vi "Collate_Measurements v0.3.vi"(1 "Collate Files":bool) -> ()   [LabVIEW 2014]
uses:
  <vilib>/Utility/error.llb/DialogType.ctl
panel:
  out "appended array":dbl[][](array[numeric])
  out "FF":dbl
  out "VOC":dbl format="%#.6g"
  out "JSC":dbl
  out "PCE":dbl
  out "Array of File Paths":string[](array[string])
  out "error out":errorcluster
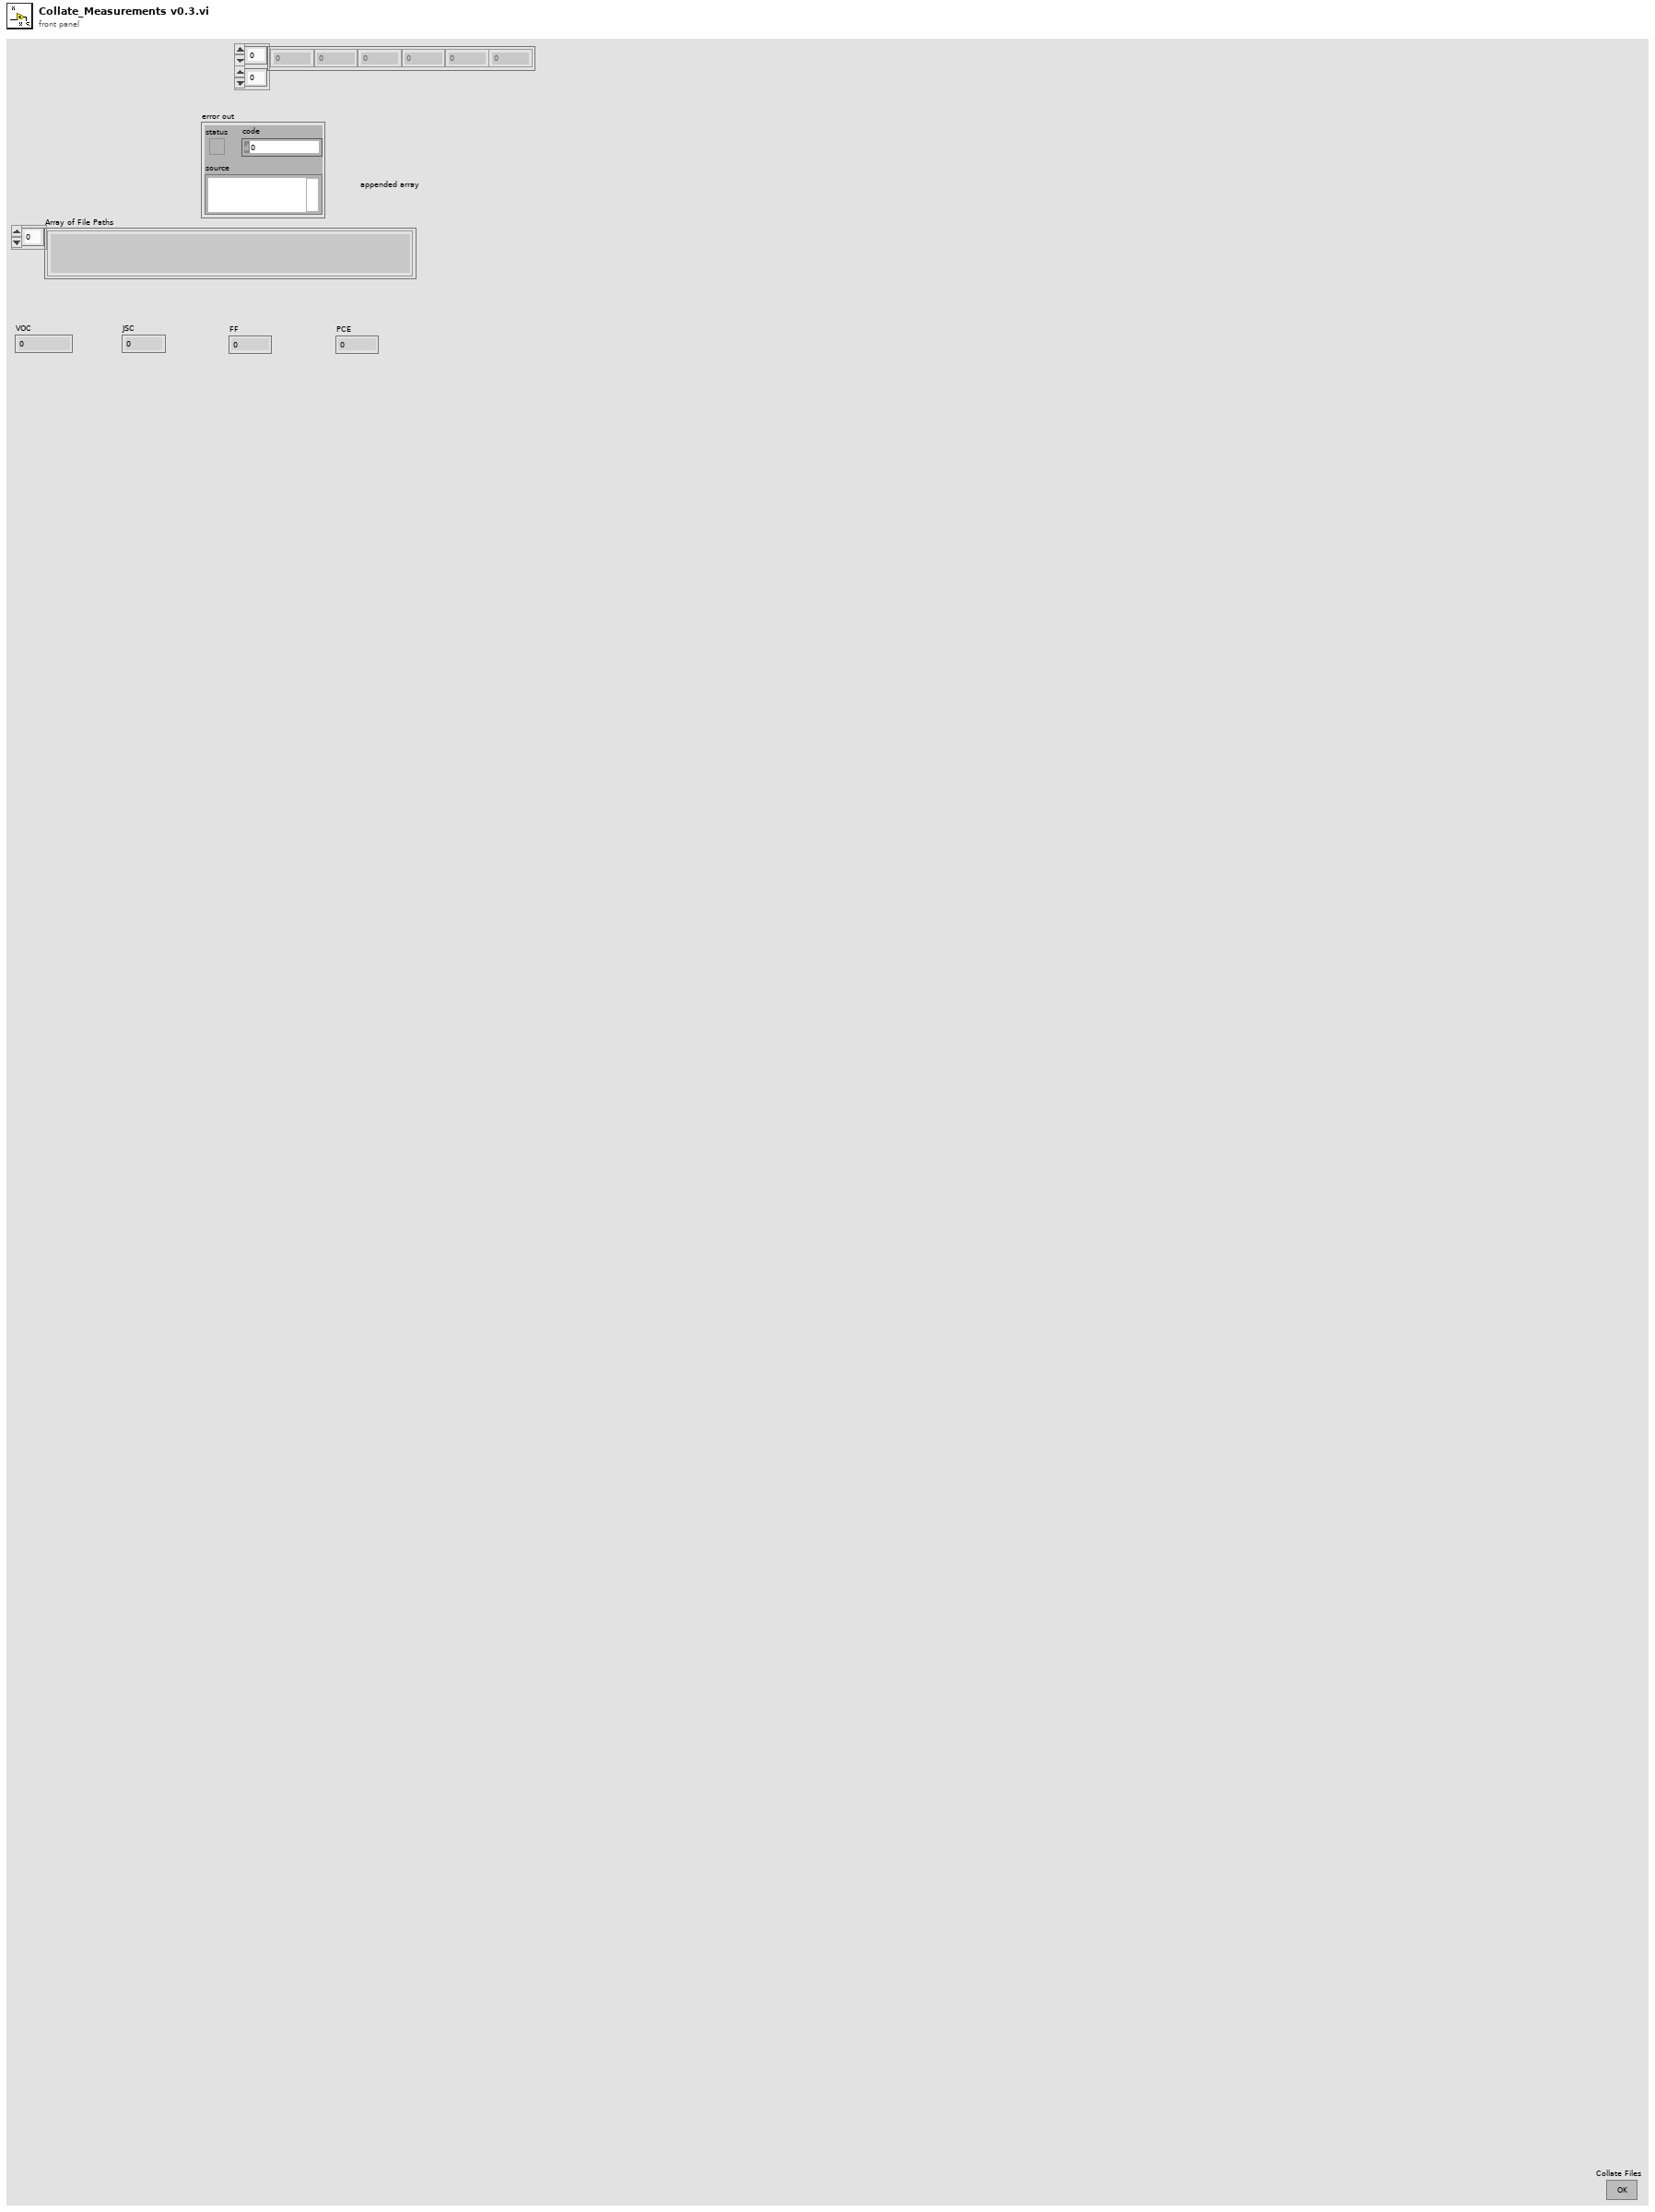
[diagram p1: front panel]
types:
  T1 = enum16{"open", "replace", "create", "open or create", "replace or create", "replace or create with confirmation"}
  T2 = typedef "DialogType.ctl" = u16
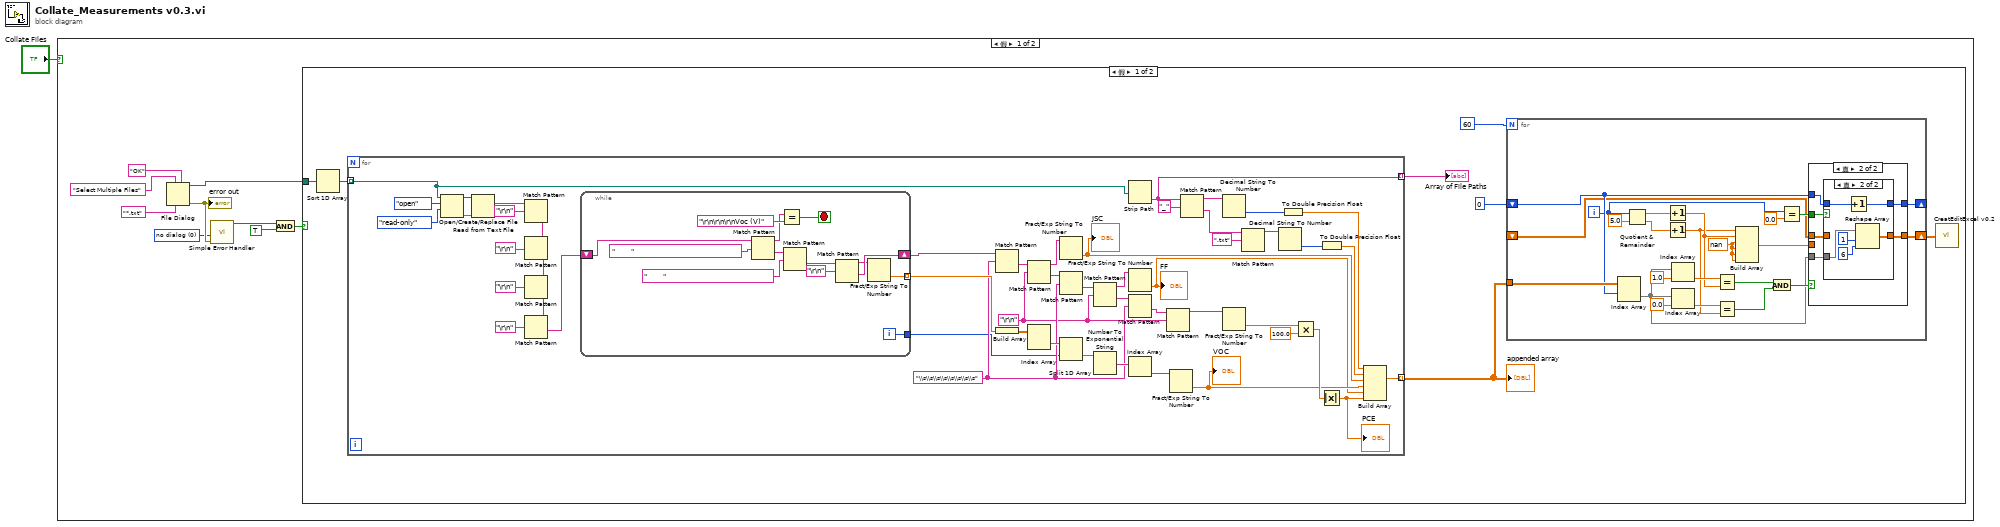
[diagram p0: block diagram]
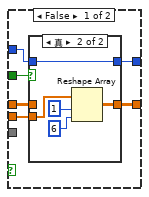
[diagram p2: hidden frame]
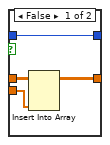
[diagram p3: hidden frame]
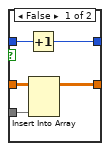
[diagram p4: hidden frame]
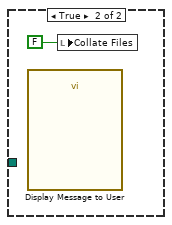
[diagram p5: hidden frame]
diagram:
  n1 = case shown="假" "Collate Files" {
    frame False {
      w2 = T2 0 items=["no dialog", "OK message", "continue or stop message", "OK message + warnings", "continue/stop + warnings"] ("type of dialog (OK msg:1)")
      n2 = File Dialog(5:"OK" ("button label"), 6:"*.txt" ("pattern (all files)"), 7:"Select Multiple Files" ("prompt")) -> (0:w6:errorcluster, 3:w7:path[])  [unwired: 1 in, 5 out]
      "error out" <- w6
      n3 = call <vilib>:"Simple Error Handler.vi"("type of dialog (OK msg:1)"=w2, "error in (no error)"=w6) -> ("error?"=w5:bool)  [unwired: 7 out]
      n4 = And(x=w5, y=TRUE) -> (x .and. y?=w3:bool)
      n5 = case shown="假" w3 {
        tunnel: w7 -> [w16 _]
        frame False {
          n6 = Sort 1D Array(array=w16) -> (sorted array=w15:path[])
          n7 = for {
            tunnel: w15 -> [w88] mode=indexing
            tunnel: [w82] -> w17 mode=indexing
            tunnel: [w73] -> w13 mode=indexing
            w97 = "\r\n"
            w99 = "\\s\\s\\s\\s\\s\\s\\s\\s" ("regular expression")
            n8 = Open/Create/Replace File(file path (use dialog)=w88, operation (0:open)=T1."open", access (0:read/write)=enum16{"read/write", "read-only", "write-only"}."read-only") -> (refnum out=w120:refnum<file>, error out=w119:errorcluster)  [unwired: 1 in, 3 out]
            n9 = Read from Text File(file (use dialog)=w120, error in=w119) -> (text=w118:string)  [unwired: 5 out]
            n10 = Match Pattern(string=w118, regular expression="\r\n") -> (after substring=w114:string)  [unwired: 4 out]
            n11 = Match Pattern(string=w114, regular expression="\r\n") -> (after substring=w113:string)  [unwired: 4 out]
            n12 = Match Pattern(string=w113, regular expression="\r\n") -> (after substring=w111:string)  [unwired: 4 out]
            n13 = Match Pattern(string=w111, regular expression="\r\n") -> (after substring=w110:string)  [unwired: 4 out]
            n14 = while {
              shift-right: [w129] -> w104
              shift-left: w110 -> [w130]
              tunnel: [w126] -> w107 mode=indexing
              tunnel: [w123] -> w89
              i -> [w123]
              stop <- w128 stop-if-true
              n15 = Match Pattern(string=w130, regular expression="        ") -> (before substring=w124:string, after substring=w135:string)  [unwired: 3 out]
              n16 = Equal?(x=w124, y="\r\n\r\n\r\nVoc (V)") -> (x = y?=w128:bool)
              n17 = Match Pattern(string=w135, regular expression="        ") -> (after substring=w134:string)  [unwired: 4 out]
              n18 = Match Pattern(string=w134, regular expression="\r\n") -> (before substring=w127:string, after substring=w129:string)  [unwired: 3 out]
              n19 = Fract/Exp String To Number(string=w127) -> (number=w126:dbl)  [unwired: 4 out]
            }
            n20 = Match Pattern(string=w104, regular expression=w99) -> (after substring=w103:string)  [unwired: 4 out]
            n21 = Build Array(w107) -> (w109:dbl[][])
            n22 = Match Pattern(string=w103, regular expression=w97) -> (before substring=w95:string, after substring=w102:string)  [unwired: 3 out]
            n23 = Index Array(array=w109) -> (element=w108:dbl[])  [unwired: 2 in]
            n24 = Fract/Exp String To Number(string=w95) -> (number=w87:dbl)  [unwired: 4 out]
            "JSC" <- w87
            n25 = Match Pattern(string=w102, regular expression=w99) -> (after substring=w101:string)  [unwired: 4 out]
            n26 = Split 1D Array(array=w108, index=w89) -> (second subarray=w106:dbl[])  [unwired: 1 out]
            n27 = Match Pattern(string=w101, regular expression=w97) -> (before substring=w94:string, after substring=w100:string)  [unwired: 3 out]
            n28 = Number To Exponential String(number=w106) -> (E-format string=w105:string[])  [unwired: 3 out]
            n29 = Strip Path(path=w88) -> (name=w82:string)  [unwired: 1 out]
            n30 = Fract/Exp String To Number(string=w94) -> (number=w85:dbl)  [unwired: 4 out]
            "FF" <- w85
            n31 = Match Pattern(string=w100, regular expression=w99) -> (after substring=w98:string)  [unwired: 4 out]
            n32 = Index Array(array=w105) -> (element=w96:string)  [unwired: 1 in]
            n33 = Match Pattern(string=w98, regular expression=w97) -> (before substring=w93:string)  [unwired: 4 out]
            n34 = Fract/Exp String To Number(string=w96) -> (number=w86:dbl)  [unwired: 4 out]
            "VOC" <- w86
            n35 = Match Pattern(string=w82, regular expression="_") -> (before substring=w79:string, after substring=w80:string)  [unwired: 3 out]
            n36 = Decimal String To Number(string=w79) -> (number=w78:i32)  [unwired: 3 out]
            n37 = Fract/Exp String To Number(string=w93) -> (number=w91:dbl)  [unwired: 4 out]
            n38 = Match Pattern(string=w80, regular expression=".txt") -> (before substring=w76:string)  [unwired: 4 out]
            n39 = Decimal String To Number(string=w76) -> (number=w75:i32)  [unwired: 3 out]
            n40 = To Double Precision Float(number=w78) -> (double precision float=w77:dbl)
            n41 = Multiply(x=w91, y=100.0) -> (x*y=w90:dbl)
            n42 = Absolute Value(x=w90) -> (abs(x)=w84:dbl)
            "PCE" <- w84
            n43 = To Double Precision Float(number=w75) -> (double precision float=w74:dbl)
            n44 = Build Array(w77, w74, w87, w86, w85, w84) -> (w73:dbl[])
          }
          "Array of File Paths" <- w17
          "appended array" <- w13
          n45 = for {
            N: 60 -> [_]
            tunnel: w13 -> [w40]
            shift-right: [w26] -> _
            shift-left: 0 ("index (row)") -> [w27]
            shift-right: [w25] -> w11
            shift-left: _ -> [w23]
            i -> [w21]
            w31 = nan ("element")
            n46 = Index Array(array=w40, index (row)=w27) -> (element=w24:dbl[])  [unwired: 1 in]
            n47 = Quotient & Remainder(x=w21, y=5.0) -> (x-y*floor(x/y)=w32:dbl, floor(x/y)=w19:dbl)
            n48 = Increment(x=w32) -> (x+1=w20:dbl)
            n49 = Increment(x=w19) -> (x+1=w18:dbl)
            n50 = Index Array(array=w24, index=1.0) -> (element=w35:dbl)
            n51 = Index Array(array=w24, index=0.0) -> (element=w36:dbl)
            n52 = Equal?(x=w35, y=w20) -> (x = y?=w34:bool)
            n53 = Equal?(x=w36, y=w18) -> (x = y?=w33:bool)
            n54 = Build Array(w18, w20, w31, w31, w31, w31) -> (w22:dbl[])
            n55 = And(x=w34, y=w33) -> (x .and. y?=w29:bool)
            n56 = Equal?(x=w21, y=0.0) -> (x = y?=w28:bool)
            n57 = case shown="真" w29 {
              tunnel: w28 -> [w43 w61]
              tunnel: w27 -> [w45 w60]
              tunnel: [w44 w59] -> w26
              tunnel: [w42 w58] -> w25
              tunnel: w24 -> [_ w57]
              tunnel: w23 -> [w41 w56]
              tunnel: w22 -> [w46 _]
              frame False {
                n58 = case shown="真" w43 {
                  tunnel: w45 -> [w47 w51]
                  tunnel: [w47 w51] -> w44
                  tunnel: [w48 w53] -> w42
                  tunnel: w46 -> [w49 w55]
                  tunnel: w41 -> [w50 _]
                  frame False {
                    n59 = Insert Into Array(array=w50, new element=w49) -> (w48:dbl[][])  [unwired: 2 in]
                  }
                  frame True {
                    n60 = Reshape Array(w55, 1 ("dimension size"), 6 ("dimension size")) -> (w53:dbl[][])
                  }
                }
              }
              frame True {
                n61 = case shown="真" w61 {
                  tunnel: w60 -> [w66 w72]
                  tunnel: [w65 w71] -> w59
                  tunnel: [w62 w68] -> w58
                  tunnel: w57 -> [w63 w70]
                  tunnel: w56 -> [w64 _]
                  frame False {
                    n62 = Increment(x=w66) -> (x+1=w65:i32)
                    n63 = Insert Into Array(array=w64, new element=w63) -> (w62:dbl[][])  [unwired: 2 in]
                  }
                  frame True {
                    n64 = Increment(x=w72) -> (x+1=w71:i32)
                    n65 = Reshape Array(w70, 1 ("dimension size"), 6 ("dimension size")) -> (w68:dbl[][])
                  }
                }
              }
            }
          }
          n66 = call "CreatEditExcel v0.2.vi"("output"=w11) -> ()  [unwired: 1 out]
        }
        frame True {
          n67 = call "Display Message to User"() -> ()  [unwired: 3 in, 9 out]
          n68 = local write "Collate Files"(FALSE ("Collate Files")) -> ()
        }
      }
    }
    frame True {
    }
  }
